vi "niFPGA BFGroup Twiddle Table 128 U32.vi"(7 "address":fxp<+,7,7>) -> (4 "twid real":fxp<+/-,17,2> format="%.16g", 6 "twid imag":fxp<+/-,17,2> format="%.16g")   [LabVIEW 2017]
uses:
  <vilib>/rvi/FXPMathLib/basic elements/FxpDiscreteDelay/XNode/nifxpmath_DiscreteDelay.xnode
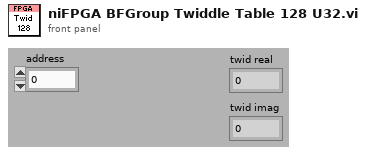
[diagram p1: front panel]
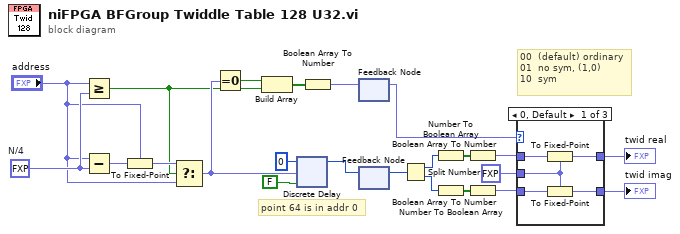
[diagram p0: block diagram]
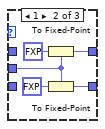
[diagram p2: hidden frame]
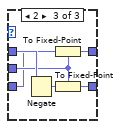
[diagram p3: hidden frame]
diagram:
  w18 = fxp<+,7,7> 64.0  # N/4
  # "point 64 is in addr 0"
  # "00  (default) ordinary\n01  no sym, (1,0)\n10  sym"
  n1 = Greater Or Equal?(x="address", y=w18) -> (x >= y?=w3:bool)
  n2 = Subtract(x="address", y=w18) -> (x-y=w17:fxp<+/-,8,8>)
  n3 = To Fixed-Point(fixed-point type="address", number=w17) -> (fixed-point=w16:fxp<+,7,7>)
  n4 = Select(t=w16, s=w3, f="address") -> (s? t:f=w6:fxp<+,7,7>)
  n5 = Equal To 0?(x=w6) -> (x = 0?=w2:bool)
  n6 = Build Array(w2, w3) -> (w4:bool[])
  n7 = xnode "Discrete Delay"("D"=u32 0, "n-1[0..63]"=w6, "enable"=FALSE) -> ("Q"=w5:u32)
  n8 = Boolean Array To Number(Boolean array=w4) -> (number=w1:fxp<+,2,2>)
  n9 = feedback-in #1(w1) -> ()
  n10 = feedback #1() -> (w9:fxp<+,2,2>)  [unwired: 1 out]
  n11 = feedback-in #2(w5) -> ()
  n12 = feedback #2() -> (w19:u32)  [unwired: 1 out]
  n13 = Split Number(x=w19) -> (hi(x)=w22:u16, lo(x)=w20:u16)
  n14 = Number To Boolean Array(number=w22) -> (Boolean array=w23:bool[])
  n15 = Number To Boolean Array(number=w20) -> (Boolean array=w21:bool[])
  n16 = Boolean Array To Number(Boolean array=w23) -> (number=w13:fxp<+/-,16,1>)
  n17 = Boolean Array To Number(Boolean array=w21) -> (number=w12:fxp<+/-,16,1>)
  n18 = case shown="0, Default" w9 {
    tunnel: w13 -> [w28 _ w39]
    tunnel: [w27 w32 w34] -> w11
    tunnel: w12 -> [w26 _ w35]
    tunnel: [w25 w30 w38] -> w10
    tunnel: fxp<+/-,17,2> 0.0 ("fixed-point type") -> [w24 w29 w36]
    frame 0, Default {
      n19 = To Fixed-Point(fixed-point type=w24, number=w28) -> (fixed-point=w27:fxp<+/-,17,2>)
      n20 = To Fixed-Point(fixed-point type=w24, number=w26) -> (fixed-point=w25:fxp<+/-,17,2>)
    }
    frame 1 {
      n21 = To Fixed-Point(fixed-point type=w29, number=fxp<+,1,1> 1.0 ("fixed-point type")) -> (fixed-point=w32:fxp<+/-,17,2>)
      n22 = To Fixed-Point(fixed-point type=w29, number=fxp<+,1,1> 0.0 ("fixed-point type")) -> (fixed-point=w30:fxp<+/-,17,2>)
    }
    frame 2 {
      n23 = Negate(x=w39) -> (-x=w37:fxp<+/-,17,2>)
      n24 = To Fixed-Point(fixed-point type=w36, number=w35) -> (fixed-point=w34:fxp<+/-,17,2>)
      n25 = To Fixed-Point(fixed-point type=w36, number=w37) -> (fixed-point=w38:fxp<+/-,17,2>)
    }
  }
  "twid real" <- w11
  "twid imag" <- w10
